vi "startSerial.vi"(8 "error in (no error)":errorcluster, 11 "TemperatureSensor in":refnum<class "TemperatureSensor.lvclass">) -> (0 "error out":errorcluster, 3 "TemperatureSensor out":refnum<class "TemperatureSensor.lvclass">)   [LabVIEW 2013, in "TemperatureSensor.lvlib" / "TemperatureSensor.lvclass"]
uses:
  <userlib>/Common/Devices/TemperatureSensor/TemperatureSensor/TemperatureSensor.lvclass
  <userlib>/Common/Devices/TemperatureSensor/TemperatureSensor/TemperatureSensor.lvclass/TemperatureSensor.ctl
  <userlib>/Common/SerialProtocols/SerialCommunicator/SerialCommunicator.lvclass
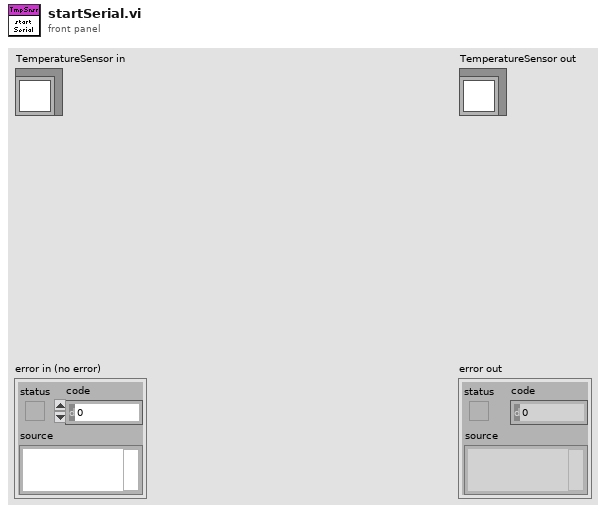
[diagram p1: front panel]
types:
  T1 = typedef "SerialProtocols.lvlib/SerialConfig.ctl" = cluster{"Serial Protocol":T2, "Protocol Parameters":T3, "Serial Message Parameters":T4}
  T2 = typedef "SerialProtocols.lvlib/SerialProtocol.ctl" = enum16{"RS232", "RS485", "SerialSimulator"}
  T3 = typedef "SerialProtocols.lvlib/ProtocolParameters.ctl" = cluster{"VISA resource name":refnum<visa-resource-name>, "Baud Rate":u32, "Data Bits":u16, "Parity":enum16{"None", "Odd", "Even", "Mark", "Space"}, "Flow Control":u16, "Stop Bits":u16, "Timeout (ms)":u32}
  T4 = typedef "SerialProtocols.lvlib/SerialMessageParameters.ctl" = cluster{"Byte Count":u32, "Enable Termination Character":bool, "Termination Char":u8}
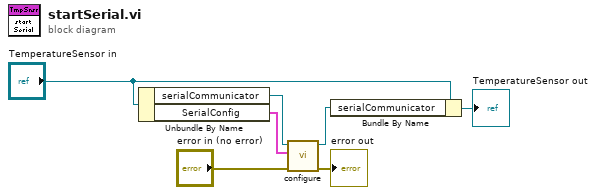
[diagram p0: block diagram]
diagram:
  n1 = Unbundle By Name("TemperatureSensor in") -> ("serialCommunicator"=w7:refnum<class "SerialCommunicator.lvclass">, "SerialConfig"=w6:T1)
  n2 = call-dynamic "configure.vi"("error in (no error)"="error in (no error)", "SerialConfig"=w6, "SerialCommunicator in"=w7) -> ("error out"=→"error out":errorcluster, "SerialCommunicator out"=w5:refnum<class "SerialCommunicator.lvclass">)  [unwired: 7 in]
  n3 = Bundle By Name(cluster="TemperatureSensor in", "serialCommunicator"=w5) -> (→"TemperatureSensor out":refnum<class "TemperatureSensor.lvclass">)
